vi "Update Cooker Duration.vi"(8 "error in (no error)":errorcluster, 10 "Duration (s)":dbl format="%.2f s", 11 "Cooker Messaging Interface in":refnum<class "Cooker Messaging Interface.lvclass">) -> (0 "error out":errorcluster, 3 "Cooker Messaging Interface out":refnum<class "Cooker Messaging Interface.lvclass">)   [LabVIEW 2021, in "Cooker Messaging Interface.lvlib" / "Cooker Messaging Interface.lvclass"]
uses:
  Cooker Messaging Interface.lvclass
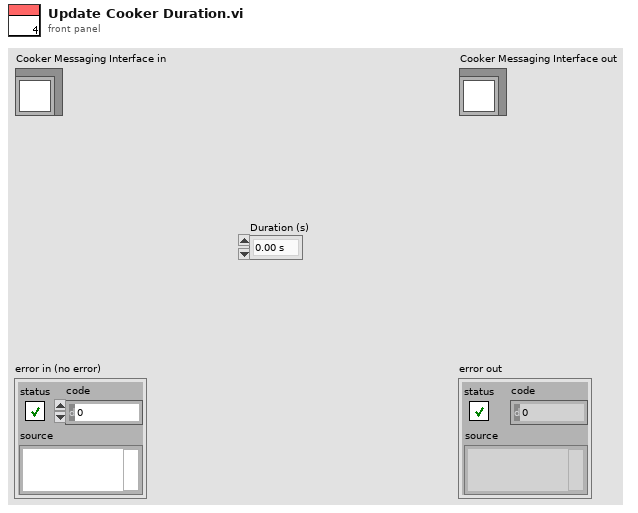
[diagram p1: front panel]
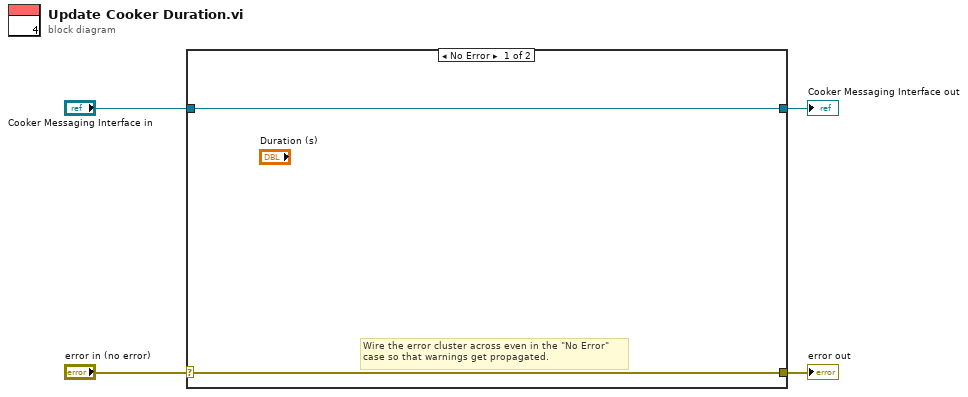
[diagram p0: block diagram]
diagram:
  n1 = case shown="No Error" "error in (no error)" {
    selector: "error in (no error)" -> [w5 w8]
    tunnel: [w5 w8] -> w3
    tunnel: [w6 w7] -> w1
    tunnel: "Cooker Messaging Interface in" -> [w6 w7]
    frame No Error {
      # "Wire the error cluster across even in the \"No Error\"\ncase so that warnings get propagated."
    }
    frame Error {
    }
  }
  "error out" <- w3
  "Cooker Messaging Interface out" <- w1
